vi "LSX Get Speed Poti.vi"(8 "error in (no error)":errorcluster, 10 "pbSpePoti":i32, 11 "lLSID":i32) -> (0 "error out":errorcluster, 2 "pbSpePoti out":i32, 3 "function return":i32)   [LabVIEW 2018, in "Tango.lvlib"]
doc: "TANGOAPI int TANGOCALL LSX_GetSpeedPoti (int lLSID, BOOL *pbSpePoti);"
uses:
  <userlib>/Tango/Tango.lvlib
  <userlib>/Tango/Tango_DLL.dll
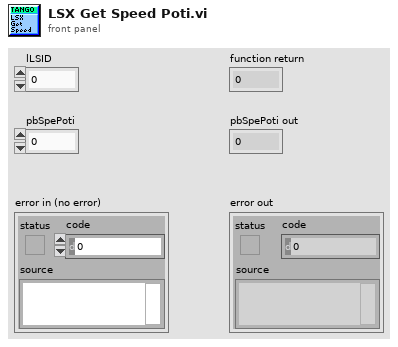
[diagram p1: front panel]
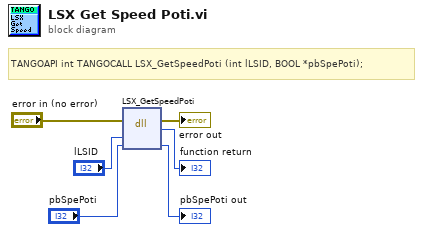
[diagram p0: block diagram]
diagram:
  # "TANGOAPI int TANGOCALL LSX_GetSpeedPoti (int lLSID, BOOL *pbSpePoti);"
  n1 = dll-call lib="C:/Program Files (x86)/National Instruments/LabVIEW 2018/user.lib/Tango/Tango_DLL.*" fn="LSX_GetSpeedPoti"(error in="error in (no error)", "lLSID"="lLSID", "pbSpePoti"="pbSpePoti") -> (error out=→"error out":errorcluster, →"function return":i32, "pbSpePoti"=→"pbSpePoti out":i32)  [unwired: 3 in, 1 out]
